vi "Switch_Close.vi"(8 "错误输入（无错误）":errorcluster, 11 "COM":refnum<visa-resource-name>) -> (0 "错误输出":errorcluster)   [LabVIEW 2018, in "Switch.lvlib"]
uses:
  Switch.lvlib
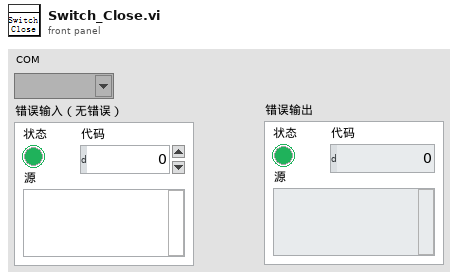
[diagram p1: front panel]
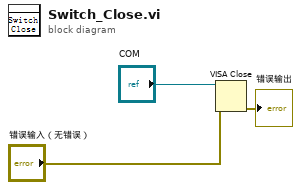
[diagram p0: block diagram]
diagram:
  n1 = VISA Close(VISA resource name="COM", error in (no error)="错误输入（无错误）") -> (error out=→"错误输出":errorcluster)
